vi "_CheckPasswordLegal.vi"(8 "error in (no error)":errorcluster, 11 "Password":string) -> (0 "error out":errorcluster, 2 "legal?":bool)   [LabVIEW 2017, in "Login-UI.lvlib"]
uses:
  Login-UI.lvlib
  <vilib>/regexp/Match Regular Expression.xnode
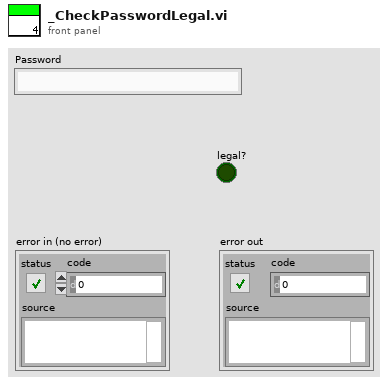
[diagram p1: front panel]
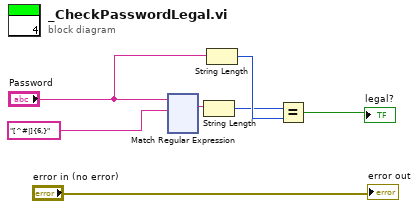
[diagram p0: block diagram]
diagram:
  n1 = xnode "Match Regular Expression"("input string"="Password", "regular expression"="[^#|]{6,}") -> ("whole match"=w2:string)  [unwired: 4 in, 4 out]
  n2 = String Length(string=w2) -> (length=w1:i32)
  n3 = String Length(string="Password") -> (length=w4:i32)
  n4 = Equal?(x=w1, y=w4) -> (x = y?=→"legal?":bool)
  "error out" <- "error in (no error)"
